vi "Get Project Refs.vi"(8 "error in":errorcluster, 10 "Target Selection":string, 11 "Project Selection":string) -> (0 "error out":errorcluster, 3 "Project":refnum<class "Project.lvclass">)   [LabVIEW 2019, in "Panther Dashboard.lvlib" / "Project.lvclass"]
uses:
  Project.lvclass
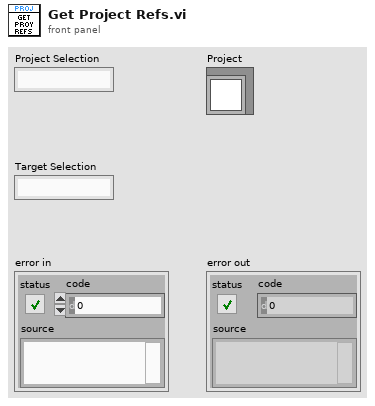
[diagram p1: front panel]
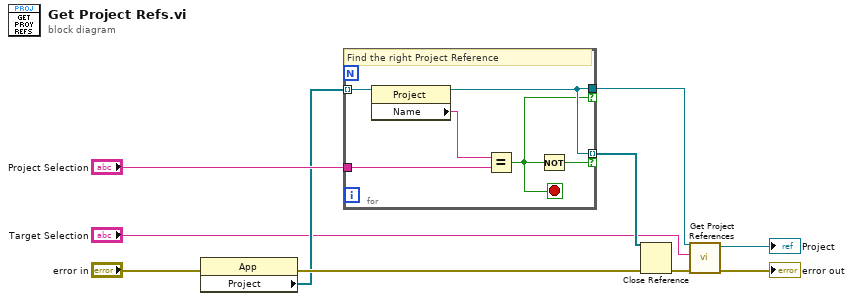
[diagram p0: block diagram]
diagram:
  n1 = property class="App"(error in="error in") -> (error out=w8:errorcluster, "Project"=w4:refnum<vi>[])  [unwired: 1 in, 1 out]
  n2 = for {
    tunnel: w4 -> [w16] mode=indexing
    tunnel: [w13] -> w5 if=w12
    tunnel: "Project Selection" -> [w14]
    tunnel: [w13] -> w3 mode=indexing if=w11
    stop <- w12 stop-if-true
    # "Find the right Project Reference"
    n3 = property class="Project"(reference=w16) -> (reference out=w13:refnum<vi>, "Name"=w15:string)  [unwired: 1 in, 1 out]
    n4 = Equal?(x=w15, y=w14) -> (x = y?=w12:bool)
    n5 = Not(x=w12) -> (.not. x?=w11:bool)
  }
  n6 = Close Reference(reference=w3, error in (no error)=w8) -> (error out=w7:errorcluster)
  n7 = call "Get Project References.vi"("error in"=w7, "Target Selection"="Target Selection", "Project in"=w5) -> ("error out"=→"error out":errorcluster, "Project"=→"Project":refnum<class "Project.lvclass">)  [unwired: 7 in]
